vi "PathPlanner_EventMarker_New.vi"(8 "Command":T1, 9 "EndPosition":dbl=-1.0, 10 "Position":dbl, 11 "TriggerName":string) -> (3 "EventMarker":T3)   [LabVIEW 2019, in "PathPlanner24.lvlib"]
doc: "Create a new event marker. This describes a position along the path that will trigger a command when reached\n\nInputs:\n - triggerName - string - The name of the trigger this event marker will control\n - position - double - The waypoint relative position of the marker\n - endPosition - double - The end waypoint relative position of the event's zone. A value of -1.0 indicates that this event is not zoned.\n - Command - cluster -- Contains the command(s) to execute. Can be null to not run a command.\n\nOutputs:\n - EventMarker - cluster - Data cluster\n\n\nNotes:\n--------\nCurrently the only type of commands that can be issued are Boolean commands. The value is forced to TRUE when the command is issued.\n\nThe following table lists the actions performed for different types of commands:\n - Unknown - nothing - not supported.\n - Wait - nothing - not supported\n - Named - Issue boolean command with TRUE value using the \"name\" as the command name.\n - Path - nothing - not supported\n - Sequential, Parallel, Race, Deadline - Issue boolean command with TRUE value for each of the commands contained in the \"commands\" array. The value for \"name\" is used as the command name."
uses:
  PathPlanner24.lvlib
  TypeDef/PathPlannerEventMarker.ctl
  TypeDef/PathPlannerCommandUtil.ctl
  ENum/PathPlanner_CommandUtilType_ENUM.ctl
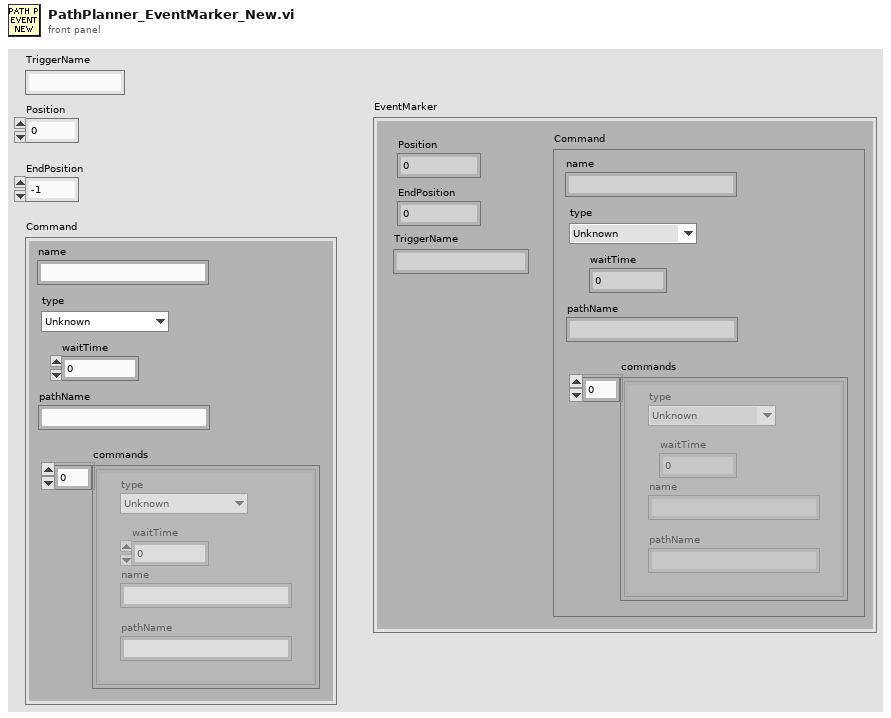
[diagram p1: front panel]
types:
  T1 = typedef "PathPlanner24.lvlib/PathPlannerCommandUtil.ctl" = cluster{"waitTime":dbl, "name":string, "pathName":string, "commands":cluster{"type":T2, "waitTime":dbl, "name":string, "pathName":string}[], "type":T2}
  T2 = typedef "PathPlanner24.lvlib/PathPlanner_CommandUtilType_ENUM.ctl" = enum16{"Unknown", "Wait", "Named", "Path", "Sequential", "Parallel", "Race", "Deadline"}
  T3 = typedef "PathPlanner24.lvlib/PathPlannerEventMarker.ctl" = cluster{"Position":dbl, "Command":T1, "TriggerName":string, "EndPosition":dbl}
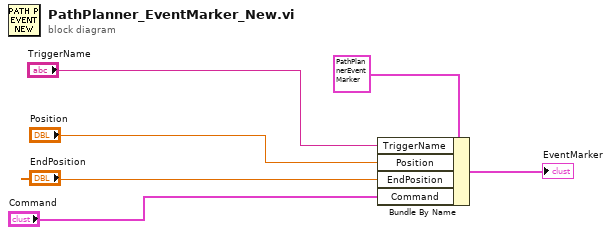
[diagram p0: block diagram]
diagram:
  n1 = Bundle By Name(cluster=T3 {"Position"=0.0, "Command"={"waitTime"=0.0, "name"="", "pathName"="", "commands"=[], "type"=enum."Unknown"}, "TriggerName"="", "EndPosition"=0.0} ("EventMarker"), "TriggerName"="TriggerName", "Position"="Position", "EndPosition"="EndPosition", "Command"="Command") -> (→"EventMarker":T3)
